vi "Send Actuator Setpoint.vi"(8 "error in (no error)":errorcluster, 11 "Model in":refnum<class "Model.lvclass">) -> (0 "error out":errorcluster, 3 "Model out":refnum<class "Model.lvclass">)   [LabVIEW 2016, in "Model.lvclass"]
uses:
  Model.lvclass
  Common_RT_FAILC/FAILC/FAILC.lvclass
  Modbus/DesktopModbus/DesktopModbus.lvclass
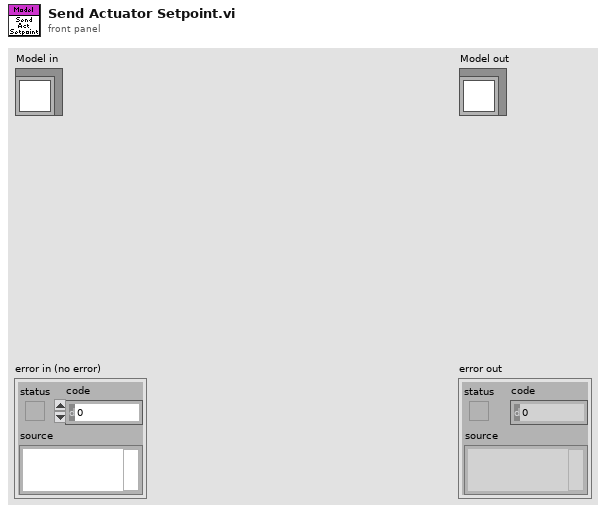
[diagram p1: front panel]
types:
  T1 = typedef "RTFAILC.lvlib/FAData.ctl" = cluster{"Constants":T2, "Command":T3, "Telemetry":T5, "Responses":T6, "Timings":T8}
  T2 = typedef "RTFAILC.lvlib/FAConstants.ctl" = cluster{"ID":i16}
  T3 = typedef "RTFAILC.lvlib/FACommand.ctl" = cluster{"AxialSetPoint":i32, "LateralSetPoint":i32, "PressureServoValveSettings":T4, "BoosterValveSettings":T4}
  T4 = typedef "RTFAILC.lvlib/FAPID.ctl" = cluster{"Kp":sgl, "Ki":sgl, "Kd":sgl, "Kf":sgl}
  T5 = typedef "RTFAILC.lvlib/FATelemetry.ctl" = cluster{"ILCFault":bool, "BroadcastCounter":u8, "AxialLoadCellForce":sgl, "LateralLoadCellForce":sgl, "AxialPressure":T4, "AxialTurbo":T4, "LateralPressure":T4, "LateralTurbo":T4}
  T6 = typedef "RTFAILC.lvlib/FAResponses.ctl" = cluster{"PIDParameters":T7, "ReadPIDParameters":T7, "SetForce":T7, "ForceAndStatus":T7}
  T7 = typedef "RTModbus.lvlib/ExceptionCodes.ctl" = u16
  T8 = typedef "RTFAILC.lvlib/FATimings.ctl" = cluster{"BroadcastSetForce":u32, "PIDParameters":u32, "FreezeSensorValues":u32, "ForceAndStatus":u32, "ReadPIDParameters":u32, "SetForce":u32}
  T9 = typedef "RTModbus.lvlib/TxFrame.ctl" = cluster{"Data":u8[], "WaitForTrigger":bool, "WaitForRx":u16, "TriggerIRQ":bool, "DelayMicroseconds":u16, "DelayMilliseconds":u16, "Timestamp":bool}
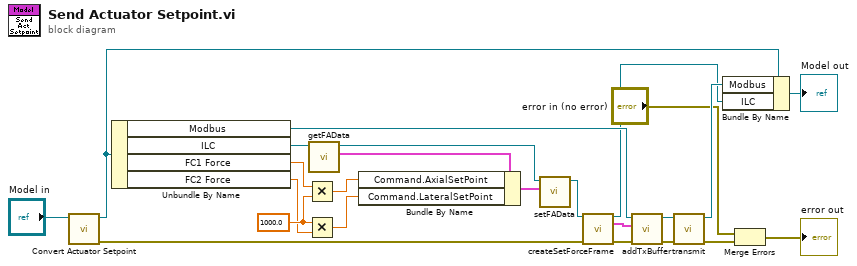
[diagram p0: block diagram]
diagram:
  w20 = 1000.0 ("y")
  n1 = call "Convert Actuator Setpoint.vi"("Model in"="Model in") -> ("error out"=w1:errorcluster, "Model out"=w2:refnum<class "Model.lvclass">)  [unwired: 9 in]
  n2 = Unbundle By Name(w2) -> ("Modbus"=w12:refnum<class "DesktopModbus.lvclass">, "ILC"=w15:refnum<class "FAILC.lvclass">, "FC1 Force"=w22:dbl, "FC2 Force"=w19:dbl)
  n3 = Multiply(x=w22, y=w20) -> (x*y=w21:dbl)
  n4 = Multiply(x=w20, y=w19) -> (x*y=w18:dbl)
  n5 = call "getFAData.vi"("FAILC in"=w15) -> ("FAData"=w23:T1, "FAILC out"=w16:refnum<class "FAILC.lvclass">)  [unwired: 9 in]
  n6 = Bundle By Name(cluster=w23, "Command.AxialSetPoint"=w21, "Command.LateralSetPoint"=w18) -> (w17:T1)
  n7 = call "setFAData.vi"("FAData"=w17, "FAILC in"=w16) -> ("FAILC out"=w14:refnum<class "FAILC.lvclass">)  [unwired: 9 in]
  n8 = call-dynamic "createSetForceFrame.vi"("FAILC in"=w14, "error in (no error)"=w1) -> ("FAILC out"=w7:refnum<class "FAILC.lvclass">, "TxFrame"=w11:T9, "error out"=w10:errorcluster)  [unwired: 11 in]
  n9 = call-dynamic "addTxBuffer.vi"("error in (no error)"=w10, "Frame"=w11, "DesktopModbus in"=w12) -> ("error out"=w9:errorcluster, "DesktopModbus out"=w13:refnum<class "DesktopModbus.lvclass">)  [unwired: 7 in]
  n10 = call-dynamic "transmit.vi"("error in (no error)"=w9, "DesktopModbus in"=w13) -> ("error out"=w6:errorcluster, "DesktopModbus out"=w8:refnum<class "DesktopModbus.lvclass">)  [unwired: 8 in]
  n11 = Bundle By Name(cluster=w2, "Modbus"=w8, "ILC"=w7) -> (→"Model out":refnum<class "Model.lvclass">)
  n12 = Merge Errors("error in (no error)", w6) -> (→"error out":errorcluster)
